vi "OnResize2.vi"(0 "XRef":T9, 1 "Bounds":T7, 2 "Mouse Mods":T5, 3 "State In":T1) -> (14 "Reply":T3, 15 "Fatal Error Out":T2, 16 "State Out":T1)   [LabVIEW 2015, in "Get Object Parameters.xnode"]
uses:
  Get Object Parameters.xnode
  <vilib>/XNodeSupport/XNodeXNodeRef.ctl
  <vilib>/XNodeSupport/XNodeRect32.ctl
  <vilib>/XNodeSupport/XNodeInt.ctl
  <vilib>/XNodeSupport/XNodeMouseMods.ctl
  <vilib>/XNodeSupport/XNodeBool.ctl
  State.ctl
  <vilib>/XNodeSupport/XNodeStringArray.ctl
  <vilib>/XNodeSupport/XNodeString.ctl
  <vilib>/XNodeSupport/XNodeErrorCluster.ctl
  dimensions.vi
  <vilib>/XNodeSupport/NI_XNodeSupport.lvlib
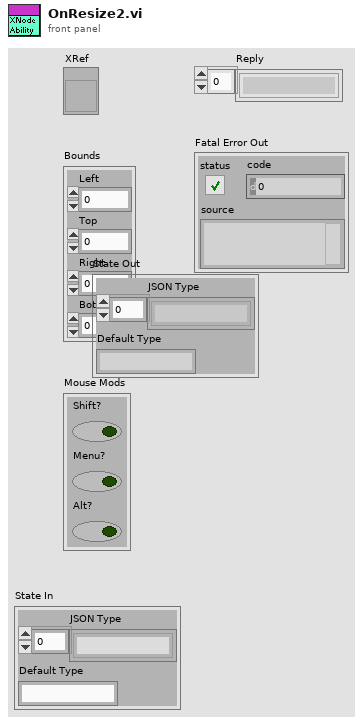
[diagram p1: front panel]
types:
  T1 = typedef "Get Object Parameters.xnode/State.ctl" = cluster{"JSON Type":string[], "Default Type":string}
  T2 = typedef "NI_XNodeSupport.lvlib/XNodeErrorCluster.ctl" = errorcluster
  T3 = typedef "NI_XNodeSupport.lvlib/XNodeStringArray.ctl" = T4[]
  T4 = typedef "NI_XNodeSupport.lvlib/XNodeString.ctl" = string
  T5 = typedef "NI_XNodeSupport.lvlib/XNodeMouseMods.ctl" = cluster{"Shift?":T6, "Menu?":T6, "Alt?":T6}
  T6 = typedef "NI_XNodeSupport.lvlib/XNodeBool.ctl" = bool
  T7 = typedef "NI_XNodeSupport.lvlib/XNodeRect32.ctl" = cluster{"Left":T8, "Top":T8, "Right":T8, "Bottom":T8}
  T8 = typedef "NI_XNodeSupport.lvlib/XNodeInt.ctl" = i32
  T9 = typedef "NI_XNodeSupport.lvlib/XNodeXNodeRef.ctl" = refnum<vi>
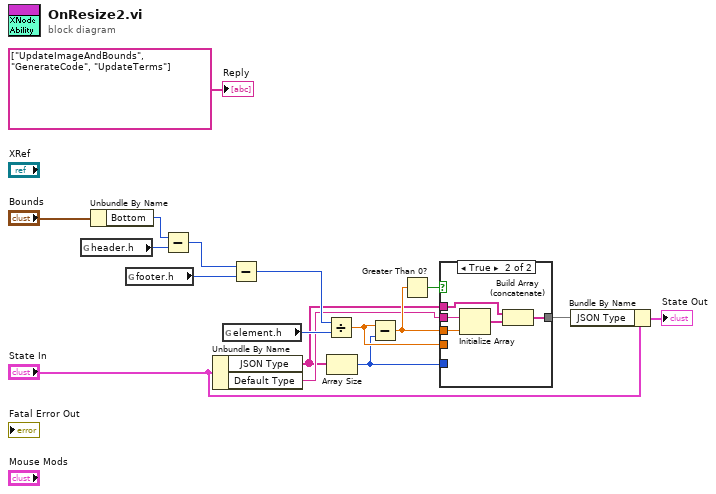
[diagram p0: block diagram]
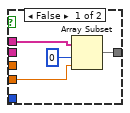
[diagram p2: hidden frame]
diagram:
  n1 = global read "dimensions.vi" "header.h"() -> (w11:i16)
  n2 = Unbundle By Name("Bounds") -> ("Bottom"=w13:T8)
  n3 = global read "dimensions.vi" "footer.h"() -> (w10:i16)
  n4 = Subtract(x=w13, y=w11) -> (x-y=w12:T8)
  n5 = Unbundle By Name("State In") -> ("JSON Type"=w2:string[], "Default Type"=w3:string)
  n6 = global read "dimensions.vi" "element.h"() -> (w14:i16)
  n7 = Subtract(x=w12, y=w10) -> (x-y=w9:T8)
  n8 = Divide(x=w9, y=w14) -> (x/y=w4:dbl)
  n9 = Array Size(array=w2) -> (size(s)=w1:i32)
  n10 = Subtract(x=w4, y=w1) -> (x-y=w6:dbl)
  n11 = Greater Than 0?(x=w6) -> (x > 0?=w7:bool)
  n12 = case shown="True" w7 {
    tunnel: w6 -> [_ w26]
    tunnel: w2 -> [w21 w25]
    tunnel: [w20 w23] -> w5
    tunnel: w1 -> [_ _]
    tunnel: w4 -> [w19 _]
    tunnel: w3 -> [_ w22]
    frame False {
      n13 = Array Subset(array=w21, index=0, length=w19) -> (w20:string[])
    }
    frame True {
      n14 = Initialize Array(w22, w26) -> (w24:string[])
      n15 = Build Array (concatenate)(w25, w24) -> (w23:string[])
    }
  }
  n16 = Bundle By Name(cluster="State In", "JSON Type"=w5) -> (→"State Out":T1)
  "Reply" <- T3 ["UpdateImageAndBounds", "GenerateCode", "UpdateTerms"] ("Reply")
